vi "plot_data_update_XY.vi"(0 "plotData":i32[][](array[numeric]), 1 "idx start":i32, 2 "length":i32, 3 "Y data":sgl[](array[numeric]) format="%.2f", 4 "X data":sgl[](array[numeric]) format="%.2f", 5 "error in (no error)":errorcluster, 6 "max value Y":sgl format="%.2f", 7 "error rangeViolation":bool=TRUE, 8 "min value Y":sgl format="%.2f", 9 "error if all equal (false)":bool, 10 "autoScale Y":bool) -> (11 "pixels Y":i32, 13 "pixels X":i32, 14 "plotData out":i32[][](array[numeric]), 15 "updated":bool, 16 "length copy":u32, 17 "dataVal max":sgl format="%.2f", 18 "dataVal min":sgl format="%.2f", 19 "error out":errorcluster)   [LabVIEW 2010, in "OSA.lvclass"]
doc: "X-data must be increasing."
uses:
  OSA.lvclass
  OSA20X_misc.lvlib
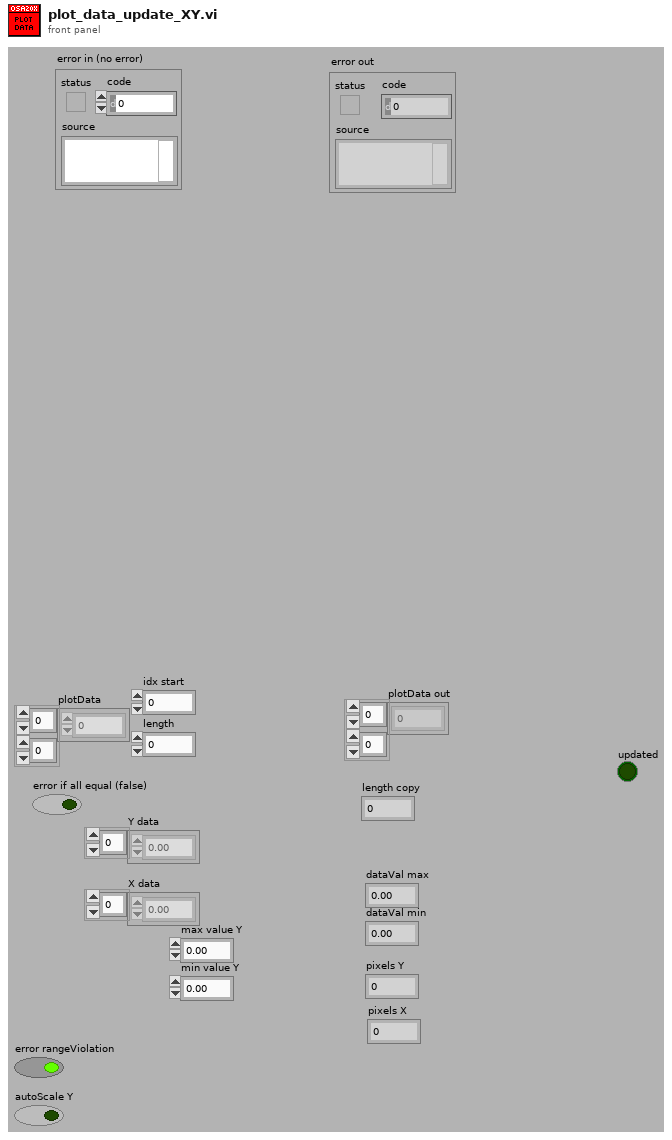
[diagram p1: front panel]
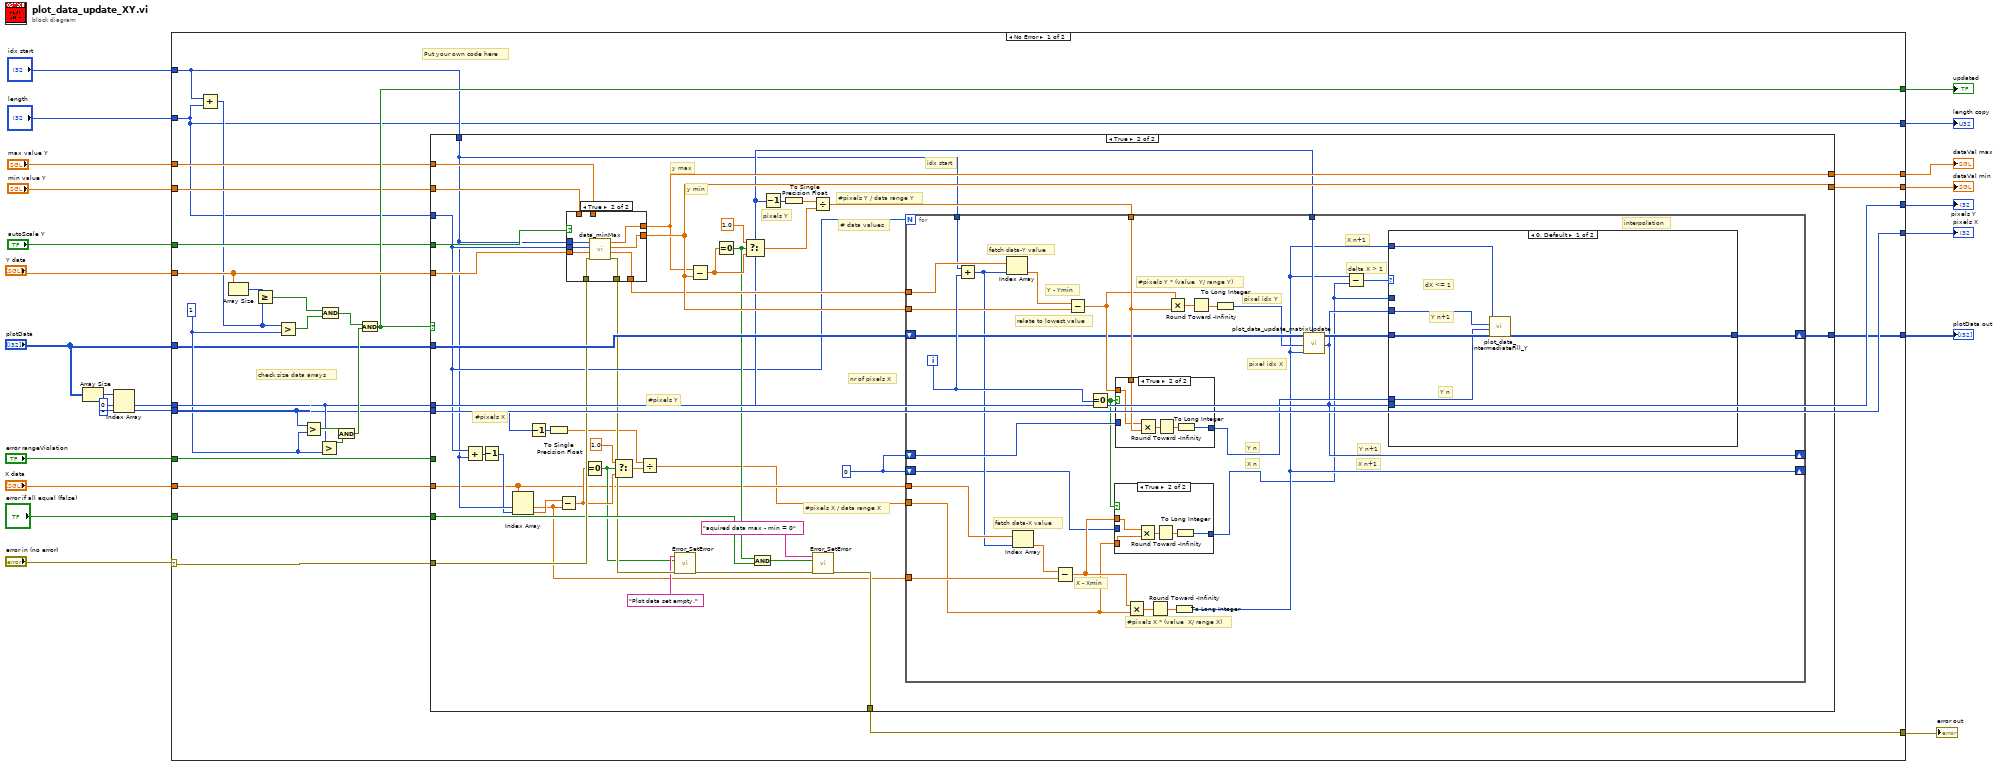
[diagram p0: block diagram]
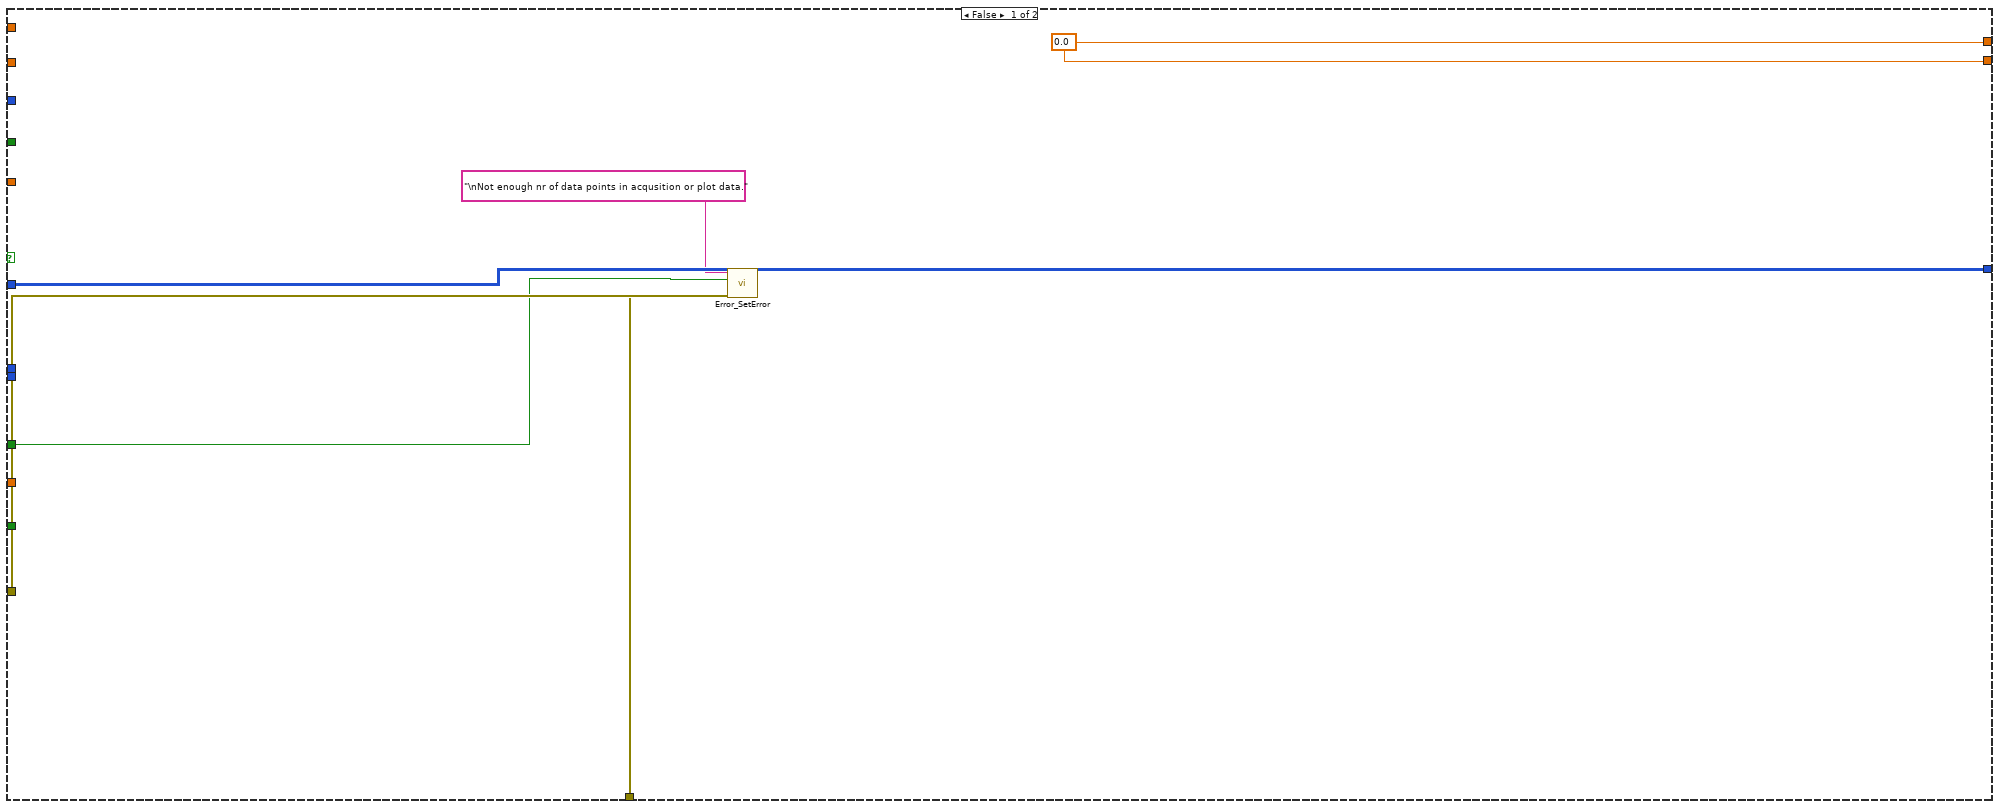
[diagram p2: hidden frame]
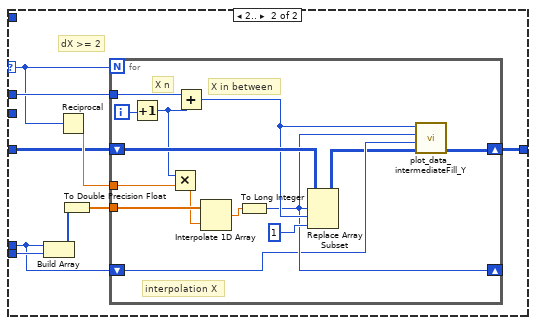
[diagram p6: hidden frame]
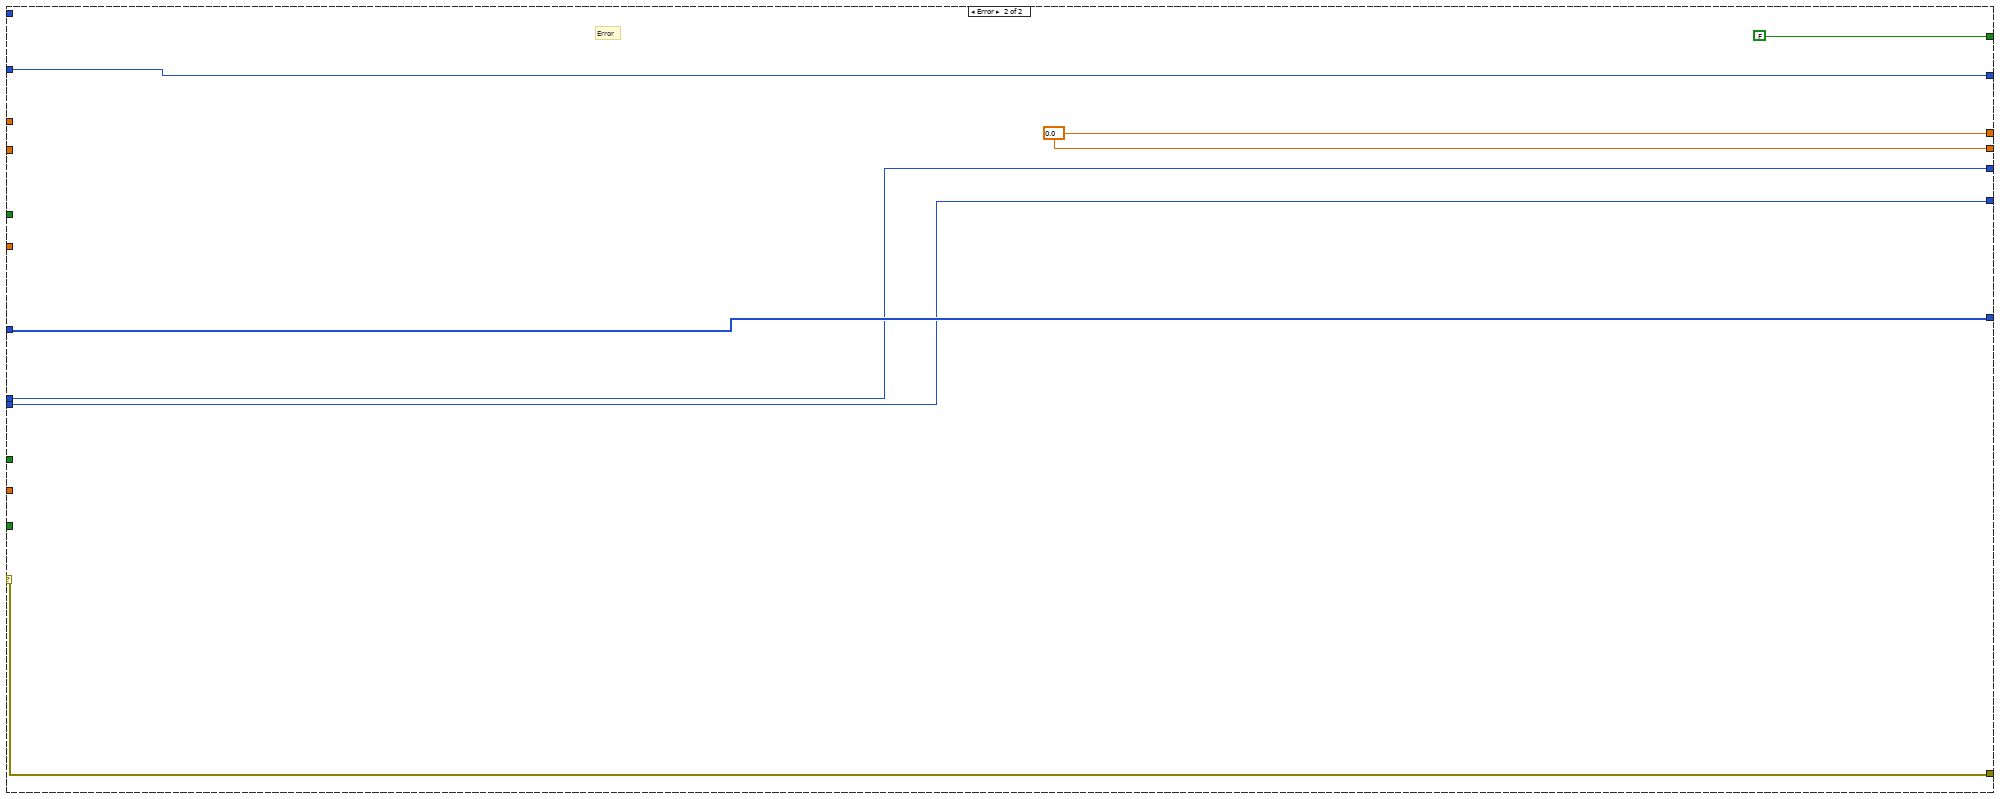
[diagram p7: hidden frame]
diagram:
  n1 = Array Size(array="plotData") -> (size(s)=w16:i32[])
  n2 = Index Array(array=w16, index #1=0 ("index"), index #2=1 ("index")) -> (element #1=w13:i32, element #2=w12:i32)
  n3 = case shown="No Error" "error in (no error)" {
    selector: "error in (no error)" -> [w42 w187]
    tunnel: [w41 w187] -> w24
    tunnel: "Y data" -> [w51 _]
    tunnel: "plotData" -> [w36 w186]
    tunnel: [w35 w186] -> w3
    tunnel: [w40 w185] -> w21
    tunnel: [w39 w185] -> w20
    tunnel: [w27 w181] -> w19
    tunnel: [w38 w184] -> w18
    tunnel: [w37 w183] -> w17
    tunnel: w13 -> [w38 w184]
    tunnel: w12 -> [w37 w183]
    tunnel: "error rangeViolation" -> [w34 _]
    tunnel: [w33 FALSE] -> w9
    tunnel: "min value Y" -> [w32 _]
    tunnel: "max value Y" -> [w31 _]
    tunnel: "autoScale Y" -> [w30 _]
    tunnel: "idx start" -> [w29 _]
    tunnel: "length" -> [w27 w181]
    tunnel: "error if all equal (false)" -> [w26 _]
    tunnel: "X data" -> [w25 _]
    frame No Error {
      w47 = u32 1 ("y")
      # "check size data arrays"
      # "Put your own code here"
      n4 = Add(x=w29, y=w27) -> (x+y=w28:i32)
      n5 = Array Size(array=w51) -> (size(s)=w50:i32)
      n6 = Greater Or Equal?(x=w50, y=w28) -> (x >= y?=w49:bool)
      n7 = Greater?(x=w28, y=w47) -> (0:w48:bool)
      n8 = Greater?(x=w37, y=w47) -> (0:w45:bool)
      n9 = Greater?(x=w38, y=w47) -> (0:w46:bool)
      n10 = And(x=w49, y=w48) -> (x .and. y?=w43:bool)
      n11 = And(x=w45, y=w46) -> (x .and. y?=w44:bool)
      n12 = And(x=w43, y=w44) -> (x .and. y?=w33:bool)
      n13 = case shown="True" w33 {
        tunnel: [w55 w98] -> w35
        tunnel: w36 -> [w55 w97]
        tunnel: w51 -> [_ w91]
        tunnel: w38 -> [_ w84]
        tunnel: w37 -> [_ w62]
        tunnel: w42 -> [w57 w92]
        tunnel: [w56 w80] -> w41
        tunnel: w27 -> [_ w73]
        tunnel: [w53 w85] -> w40
        tunnel: [w53 w93] -> w39
        tunnel: w34 -> [w52 _]
        tunnel: w32 -> [_ w96]
        tunnel: w31 -> [_ w95]
        tunnel: w30 -> [_ w94]
        tunnel: w29 -> [_ w72]
        tunnel: w26 -> [_ w78]
        tunnel: w25 -> [_ w60]
        frame False {
          w53 = sgl 0.0
          n14 = call "Error_SetError.vi"("error in"=w57, "status (true)"=w52, "source(\"\")"="\nNot enough nr of data points in acqusition or plot data." ("source(\"\")")) -> ("error out"=w56:errorcluster)  [unwired: 4 in]
        }
        frame True {
          w87 = 0
          # "#pixels X / data range X"
          # "# data values"
          # "#pixels X"
          # "#pixels Y"
          # "y min"
          # "y max"
          # "idx start"
          # "#pixels Y / data range Y"
          # "nr of pixels X"
          # "pixels Y"
          n15 = Add(x=w73, y=w72) -> (x+y=w71:i32)
          n16 = Decrement(x=w71) -> (x-1=w70:i32)
          n17 = Index Array(array=w60, index #1=w72, index #2=w70) -> (element #1=w58:sgl, element #2=w69:sgl)
          n18 = Decrement(x=w62) -> (x-1=w64:i32)
          n19 = To Single Precision Float(number=w64) -> (single precision float=w61:sgl)
          n20 = Subtract(x=w69, y=w58) -> (x-y=w74:sgl)
          n21 = case shown="True" w94 {
            tunnel: w96 -> [w101 _]
            tunnel: w95 -> [w102 _]
            tunnel: w91 -> [w100 w110]
            tunnel: [w100 w109] -> w86
            tunnel: [w102 w108] -> w85
            tunnel: [w101 w107] -> w93
            tunnel: w92 -> [w99 w106]
            tunnel: [w99 w105] -> w68
            tunnel: w72 -> [_ w104]
            tunnel: w73 -> [_ w103]
            frame False {
            }
            frame True {
              n22 = call "data_minMax.vi"("error in (no error)"=w106, "AcqData"=w110, "length"=w103, "idx start"=w104) -> ("error out"=w105:errorcluster, "dataOut"=w109:sgl[], "min"=w107:sgl, "max"=w108:sgl)  [unwired: 4 in]
            }
          }
          n23 = Equal To 0?(x=w74) -> (x = 0?=w65:bool)
          n24 = Select(t=sgl 1.0 ("x-y"), s=w65, f=w74) -> (s? t:f=w63:sgl)
          n25 = Divide(x=w61, y=w63) -> (x/y=w59:sgl)
          n26 = call "Error_SetError.vi"("error in"=w68, "status (true)"=w65, "source(\"\")"="Plot data set empty." ("source(\"\")")) -> ("error out"=w67:errorcluster)  [unwired: 4 in]
          n27 = Subtract(x=w85, y=w93) -> (x-y=w82:sgl)
          n28 = Equal To 0?(x=w82) -> (x = 0?=w77:bool)
          n29 = Select(t=sgl 1.0 ("x-y"), s=w77, f=w82) -> (s? t:f=w81:sgl)
          n30 = And(x=w77, y=w78) -> (x .and. y?=w76:bool)
          n31 = Decrement(x=w84) -> (x-1=w89:i32)
          n32 = To Single Precision Float(number=w89) -> (single precision float=w90:sgl)
          n33 = Divide(x=w90, y=w81) -> (x/y=w88:sgl)
          n34 = call "Error_SetError.vi"("error in"=w67, "status (true)"=w76, "source(\"\")"="aquired data max - min = 0" ("source(\"\")")) -> ("error out"=w80:errorcluster)  [unwired: 4 in]
          n35 = for {
            N: w73 -> [_]
            shift-right: [w140] -> w98
            shift-left: w97 -> [w127]
            tunnel: w86 -> [w134]
            tunnel: w88 -> [w139]
            shift-right: [w124] -> _
            shift-left: w87 -> [w138]
            shift-right: [w116] -> _
            shift-left: w87 -> [w112]
            tunnel: w93 -> [w130]
            tunnel: w72 -> [w132]
            tunnel: w84 -> [w123]
            tunnel: w60 -> [w122]
            tunnel: w59 -> [w113]
            tunnel: w58 -> [w119]
            i -> [w133]
            # "#pixels X * (value  X/ range X)"
            # "Y - Ymin"
            # "X - Xmin"
            # "fetch data-X value"
            # "X n+1"
            # "#pixels Y * (value  Y/ range Y)"
            # "relate to lowest value"
            # "fetch data-Y value"
            # "X n"
            # "Y n"
            # "pixel idx X"
            # "pixel idx Y"
            # "delta X > 1"
            # "interpolation"
            # "Y n+1"
            # "X n+1"
            n36 = Add(x=w132, y=w133) -> (x+y=w121:i32)
            n37 = Index Array(array=w134, index=w121) -> (element=w131:sgl)
            n38 = Index Array(array=w122, index=w121) -> (element=w120:sgl)
            n39 = Subtract(x=w120, y=w119) -> (x-y=w114:sgl)
            n40 = Subtract(x=w131, y=w130) -> (x-y=w135:sgl)
            n41 = Equal To 0?(x=w133) -> (x = 0?=w115:bool)
            n42 = case shown="True" w115 {
              tunnel: w113 -> [_ w144]
              tunnel: w114 -> [_ w143]
              tunnel: [w141 w142] -> w111
              tunnel: w112 -> [w141 _]
              frame False {
              }
              frame True {
                n43 = Multiply(x=w143, y=w144) -> (x*y=w145:sgl)
                n44 = Round Toward -Infinity(1:w145) -> (0:w146:sgl)
                n45 = To Long Integer(number=w146) -> (32bit integer=w142:i32)
              }
            }
            n46 = case shown="True" w115 {
              tunnel: w139 -> [_ w150]
              tunnel: w135 -> [_ w149]
              tunnel: [w147 w148] -> w136
              tunnel: w138 -> [w147 _]
              frame False {
              }
              frame True {
                n47 = Multiply(x=w149, y=w150) -> (x*y=w151:sgl)
                n48 = Round Toward -Infinity(1:w151) -> (0:w152:sgl)
                n49 = To Long Integer(number=w152) -> (32bit integer=w148:i32)
              }
            }
            n50 = Multiply(x=w114, y=w113) -> (x*y=w118:sgl)
            n51 = Round Toward -Infinity(1:w118) -> (0:w117:sgl)
            n52 = Multiply(x=w135, y=w139) -> (x*y=w129:sgl)
            n53 = To Long Integer(number=w117) -> (32bit integer=w116:i32)
            n54 = Round Toward -Infinity(1:w129) -> (0:w128:sgl)
            n55 = To Long Integer(number=w128) -> (32bit integer=w125:i32)
            n56 = call "plot_data_update_matrixUpdate.vi"("XY plot"=w127, "idx Y"=w125, "idx X"=w116, "Y size"=w123) -> ("XY plot out"=w126:i32[][], "idx Y out"=w124:i32)  [unwired: 13 in, 1 out]
            n57 = Subtract(x=w116, y=w111) -> (x-y=w137:i32)
            n58 = case shown="0, Default" w137 {
              selector: w137 -> [_ w158]
              tunnel: w136 -> [w154 w160]
              tunnel: w124 -> [_ w166]
              tunnel: [w153 w163] -> w140
              tunnel: w126 -> [w156 w161]
              tunnel: w124 -> [w155 _]
              tunnel: w116 -> [w157 _]
              tunnel: w111 -> [_ w159]
              frame 0, Default {
                # "Y n"
                # "Y n+1"
                # "dX <= 1"
                n59 = call "plot_data_intermediateFill_Y.vi"("plotData"=w156, "idx Y (n)"=w154, "idx Y (n+1)"=w155, "idx X"=w157) -> ("plotData out"=w153:i32[][])  [unwired: 7 in]
              }
              frame 2.. {
                # "dX >= 2"
                n60 = Build Array(w160, w166) -> (w165:i32[])
                n61 = Reciprocal(x=w158) -> (1/x=w164:dbl)
                n62 = To Double Precision Float(number=w165) -> (double precision float=w162:dbl[])
                n63 = for {
                  N: w158 -> [_]
                  shift-right: [w168] -> w163
                  shift-left: w161 -> [w179]
                  tunnel: w159 -> [w180]
                  tunnel: w162 -> [w178]
                  tunnel: w164 -> [w175]
                  shift-right: [w171] -> _
                  shift-left: w160 -> [w170]
                  i -> [w177]
                  # "X n"
                  # "X in between"
                  # "interpolation X"
                  n64 = Increment(x=w177) -> (x+1=w176:i32)
                  n65 = Multiply(x=w176, y=w175) -> (x*y=w174:dbl)
                  n66 = Add(x=w180, y=w176) -> (x+y=w172:i32)
                  n67 = Interpolate 1D Array(1:w174, 2:w178) -> (0:w167:dbl)
                  n68 = To Long Integer(number=w167) -> (32bit integer=w171:i32)
                  n69 = Replace Array Subset(array=w179, new element=1 ("new element/subarray"), index (row)=w171, index (col)=w172) -> (w169:i32[][])
                  n70 = call "plot_data_intermediateFill_Y.vi"("plotData"=w169, "idx Y (n)"=w170, "idx Y (n+1)"=w171, "idx X"=w172) -> ("plotData out"=w168:i32[][])  [unwired: 7 in]
                }
              }
            }
          }
        }
      }
    }
    frame Error {
      w185 = sgl 0.0
      # "Error"
    }
  }
  "error out" <- w24
  "plotData out" <- w3
  "dataVal max" <- w21
  "dataVal min" <- w20
  "length copy" <- w19
  "pixels Y" <- w18
  "pixels X" <- w17
  "updated" <- w9
